vi "Transducer Calibration Panel.vi"() -> ()   [LabVIEW 2015]
panel:
  out "blorp":dbl
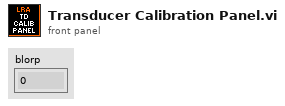
[diagram p1: front panel]
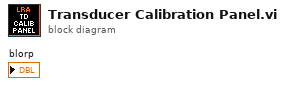
[diagram p0: block diagram]
diagram:
